vi "Framework Test.vi"() -> ()   [LabVIEW 2017]
uses:
  Builds/Data Sharing Framework/Windows/32/Data Sharing Framework Core/DSF Core.lvlibp/DSF Configuration API/Public/Controls/DSF Direction.ctl
  Builds/Data Sharing Framework/Windows/32/Data Sharing Framework Core/DSF Core.lvlibp/DSF Configuration API/Public/Controls/DSF Timing Info.ctl
  Builds/Data Sharing Framework/Windows/32/Data Sharing Framework Core/DSF Core.lvlibp/DSF Configuration API/Public/Controls/DSF Settings Info.ctl
  Builds/Data Sharing Framework/Windows/32/Data Sharing Framework Core/DSF Core.lvlibp/DSF Configuration API/Public/Controls/DSF Data Type.ctl
  <vilib>/Platform/TimedLoop/XDataNode/timing_clust.ctl
  <vilib>/Platform/TimedLoop/XDataNode/nitl_modes.ctl
  <vilib>/Platform/TimedLoop/XDataNode/wakeup.ctl
  Builds/Data Sharing Framework/Windows/32/Data Sharing Framework Core/DSF Core.lvlibp/Engine/Classes/Debug/FIFO Flags.lvclass
  Builds/Data Sharing Framework/Windows/32/Data Sharing Framework Core/DSF Core.lvlibp/Engine/Classes/Debug/Debug Flags.lvclass
  Builds/Data Sharing Framework/Windows/32/Data Sharing Framework Core/DSF Core.lvlibp/Engine/Classes/Framework/Framework.lvclass
  <vilib>/NI/Memory Manager/Classes/Pointer/Memory.Pointer.lvclass/Memory.Pointer.ctl
  <vilib>/NI/Memory Manager/Classes/Pointer/Memory.Pointer.New.4B.vi
  <vilib>/NI/Memory Manager/Classes/Pointer/Memory.Pointer.Write.0D.U32.vi
  <vilib>/NI/Memory Manager/Classes/Pointer/Memory.Pointer.New.1B.vi
  <vilib>/NI/Memory Manager/Classes/Pointer/Memory.Pointer.Write.0D.Bool.vi
  <vilib>/NI/Memory Manager/Classes/Pointer/Memory.Pointer.New.8B.vi
  <vilib>/NI/Memory Manager/Classes/Pointer/Memory.Pointer.Read.0D.I32.vi
  <vilib>/NI/Memory Manager/Classes/Pointer/Memory.Pointer.Read.0D.U32.vi
  <vilib>/NI/Memory Manager/Classes/Pointer/Memory.Pointer.Read.0D.Bool.vi
  <vilib>/NI/Memory Manager/Classes/Pointer/Memory.Pointer.Write.0D.I32.vi
  <vilib>/NI/Memory Manager/Classes/Pointer/Memory.Pointer.Allocate.vi
  <vilib>/NI/Memory Manager/Classes/Pointer/Memory.Pointer.Write.No Check.0D.U32.vi
  <vilib>/NI/Memory Manager/Classes/Pointer/Memory.Pointer.Parameter Check.Null Pointer.vi
  <vilib>/NI/Memory Manager/Classes/Pointer/Memory.Pointer.Parameter Check.Subset.vi
  <vilib>/NI/Memory Manager/Classes/Pointer/Memory.Pointer.Write.No Check.0D.Bool.vi
  <vilib>/NI/Memory Manager/Classes/Pointer/Memory.Pointer.Read.No Check.0D.I32.vi
  <vilib>/NI/Memory Manager/Classes/Pointer/Memory.Pointer.Read.No Check.0D.U32.vi
  <vilib>/NI/Memory Manager/Classes/Pointer/Memory.Pointer.Read.No Check.0D.Bool.vi
  <vilib>/NI/Memory Manager/Classes/Pointer/Memory.Pointer.Write.No Check.0D.I32.vi
  <vilib>/NI/Memory Manager/Classes/Pointer/Memory.Pointer.Set Address.vi
  <vilib>/NI/Memory Manager/Classes/Pointer/Memory.Pointer.Set Size.vi
  <vilib>/NI/Memory Manager/Classes/Pointer/Memory.Pointer.Set Allocated.vi
  <vilib>/NI/Memory Manager/Classes/Pointer/Memory.Pointer.Errors.vi
  <vilib>/NI/Memory Manager/Classes/Pointer/Memory.Pointer.Errors.Null Pointer.vi
  <vilib>/NI/Memory Manager/Classes/Pointer/Memory.Pointer.Errors.Out of Bounds.vi
  <vilib>/NI/Memory Manager/Classes/Pointer/Memory.Pointer.Errors.Create Error.vi
  <vilib>/NI/Memory Manager/VIs/Source.Write.String.vi
  <vilib>/NI/Memory Manager/Classes/Pointer/Memory.Pointer.Errors.Write Pointer Size.vi
  <vilib>/NI/Memory Manager/VIs/Source.Write.Scalar.Base10.vi
  <vilib>/NI/Memory Manager/VIs/Source.Write.Scalar.Base10 (U64).vi
  <vilib>/NI/Memory Manager/VIs/New Error Cluster Constant.vi
  <vilib>/NI/Memory Manager/VIs/New Error Cluster Constant (512B).vi
  <vilib>/NI/Memory Manager/VIs/Error Cluster.Set Status.vi
  <vilib>/NI/Memory Manager/VIs/Error Cluster.Set Code.vi
  <vilib>/NI/Memory Manager/VIs/Error Cluster.Set VI Source.vi
  <vilib>/NI/Memory Manager/Constants/Memory.Constants.vi
  <vilib>/NI/Memory Manager/Constants/Memory.Constants.Library Name.vi
  <vilib>/NI/Memory Manager/Classes/Pointer/Memory.Pointer.Errors.Get Info.vi
  <vilib>/NI/Memory Manager/Classes/Pointer/Memory.Pointer.lvclass
  <vilib>/platform/TimedLoop/XDataNode/XDataNode.xnode
  <vilib>/Platform/TimedLoop/XDataNode/XDNodeRunTimeDep.lvlib
  Builds/Data Sharing Framework/Windows/32/Data Sharing Framework Core/DSF Core.lvlibp/Shared/Classes/Framework/Framework Configuration.lvclass
  Builds/Data Sharing Framework/Windows/32/Data Sharing Framework Core/DSF Core.lvlibp/Engine/Classes/Status/Framework Status.lvclass
  Builds/Data Sharing Framework/Windows/32/Data Sharing Framework Core/DSF Core.lvlibp/Engine/Classes/Status/Framework Performance.lvclass
  Builds/Data Sharing Framework/Windows/32/Data Sharing Framework Core/DSF Core.lvlibp
panel:
  in  "UDP Rx max size":i32=800
  in  "UDP Rx ports":u16[](array[numeric])=[60000, 60001, 60002, 60003]
  in  "Plugins":T5(array[cluster])=[{"plugin class"="UDP Transceiver", "group configs"=[{"direction"=enum."Tx", "timing"={"priority"=100, "decimation"=1, "offset"=0}, "settings"=[], "transfer configs"=[{"random types?"=FALSE, "non-random type"=enum."DBL", "channel count"=100, "settings"=[{"key"="Destination Address", "value"="localhost"}, {"key"="Destination Port", "value"="60000"}]}]}, {"direction"=enum."Tx", "timing"={"priority"=100, "decimation"=2, "offset"=0}, "settings"=[], "transfer configs"=[{"random types?"=FALSE, "non-random type"=enum."DBL", "channel count"=100, "settings"=[{"key"="Destination Address", "value"="localhost"}, {"key"="Destination Port", "value"="60001"}]}]}, {"direction"=enum."Tx", "timing"={"priority"=100, "decimation"=3, "offset"=0}, "settings"=[], "transfer configs"=[{"random types?"=FALSE, "non-random type"=enum."DBL", "channel count"=100, "settings"=[{"key"="Destination Address", "value"="localhost"}, {"key"="Destination Port", "value"="60002"}]}]}, {"direction"=enum."Tx", "timing"={"priority"=100, "decimation"=4, "offset"=0}, "settings"=[], "transfer configs"=[{"random types?"=FALSE, "non-random type"=enum."DBL", "channel count"=100, "settings"=[{"key"="Destination Address", "value"="localhost"}, {"key"="Destination Port", "value"="60003"}]}]}], "plugin timing"={"priority"=100, "decimation"=1, "offset"=0}, "settings"=[{"key"="Local Port", "value"="50000"}]}]
  in  "Infinite Timeouts":bool=TRUE
  out "Framework Error":errorcluster
  out "Tx duration":u32 format="%d us"
  out "Rx duration":u32 format="%d us"
  out "Actual Frequency":dbl format="%.0pHz"
  in  "Transceiver Count":i32=4
  in  "Configuration Path":path=path "C:/Users/Admin/Desktop/test.dsf"
  out "Framework Iteration":i32 format="%d cycles"
  out "Actual Period":u32 format="%d us"
  in  "Target PCL Period":u32=10000 caption="Target Period" format="%d us"
  in  "stop":bool
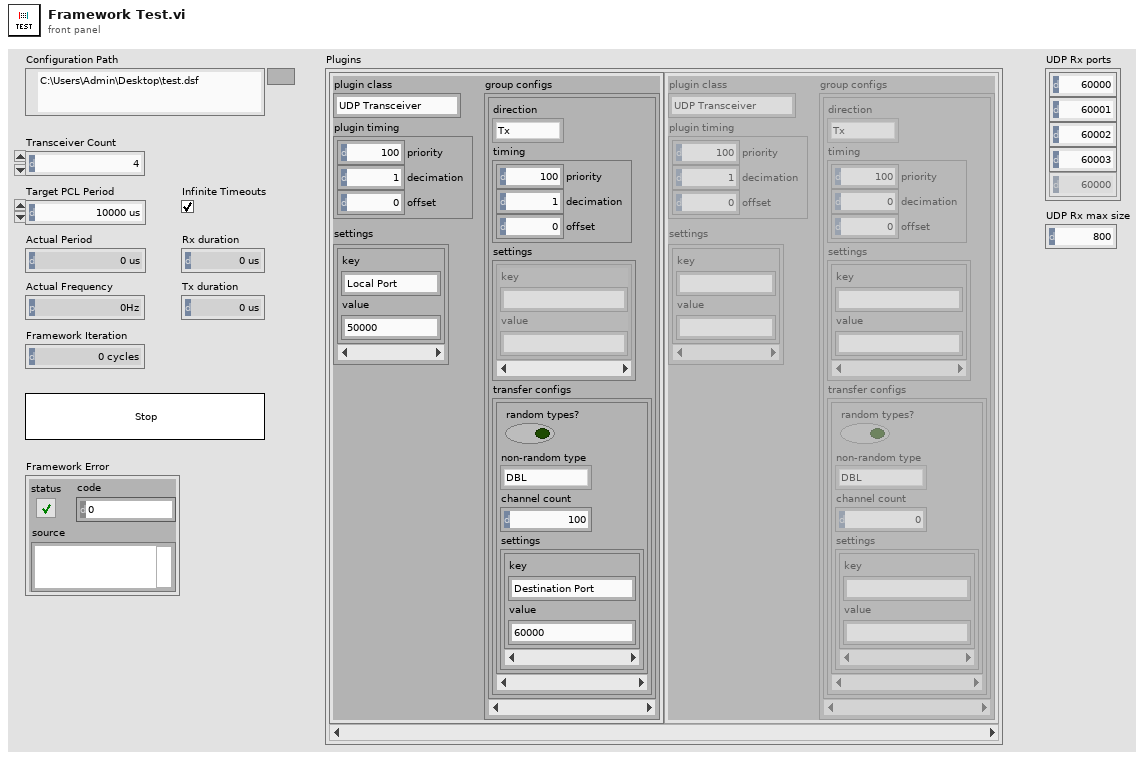
[diagram p1: front panel]
types:
  T1 = typedef "DSF Core.lvlibp/DSF Direction.ctl" = enum8{"Tx", "Rx"}
  T2 = typedef "DSF Core.lvlibp/DSF Timing Info.ctl" = cluster{"priority":u64, "decimation":u64, "offset":u64}
  T3 = typedef "DSF Core.lvlibp/DSF Settings Info.ctl" = cluster{"key":string, "value":string}[]
  T4 = typedef "DSF Core.lvlibp/DSF Data Type.ctl" = enum8{"Bool", "SGL", "DBL", "I8", "I16", "I32", "I64", "U8", "U16", "U32", "U64"}
  T5 = cluster{"plugin class":string, "group configs":cluster{"direction":T1, "timing":T2, "settings":T3, "transfer configs":cluster{"random types?":bool, "non-random type":T4, "channel count":i32, "settings":T3}[]}[], "plugin timing":T2, "settings":T3}[]
  T6 = typedef "DSF Core.lvlibp/DSF Engine Framework Configuration.ctl" = cluster{"Plugins":T7[]}
  T7 = typedef "DSF Core.lvlibp/DSF Engine Plugin Configuration.ctl" = cluster{"name":string, "class":string, "cycle timing":T2, "Transfer Groups":T8[], "settings":T3}
  T8 = typedef "DSF Core.lvlibp/DSF Engine Transfer Group Configuration.ctl" = cluster{"name":string, "direction":T1, "cycle timing":T2, "Transfers":T9[], "settings":T3}
  T9 = typedef "DSF Core.lvlibp/DSF Engine Transfer Configuration.ctl" = cluster{"name":string, "byte order":T10, "channel configurations":T11[], "settings":T3}
  T10 = typedef "DSF Core.lvlibp/DSF Byte Order.ctl" = enum8{"big-endian", "little-endian"}
  T11 = typedef "DSF Core.lvlibp/DSF Engine Channel Configuration.ctl" = cluster{"engine offset":u64, "name":string, "data type":T4, "count":u64, "buffer offset":u64, "settings":T3}
  T12 = typedef "XDNodeRunTimeDep.lvlib/timing_clust.ctl" = cluster{"Expected End [f-1]":u64, "Actual End [f-1]":u64, "Finished Late? [f-1]":bool, "Expected End [i-1]":u64, "Actual End [i-1]":u64, "Finished Late? [i-1]":bool, "Expected Start [i]":u64, "Actual Start [i]":u64, "Expected Start [f]":u64, "Actual Start [f]":u64, "Source Name":string, "Structure Name":string, "Period":i64, "Deadline":i64, "Offset":i64, "Start":i64, "Priority":i32, "Timeout":i32, "Mode":T13, "Wakeup Reason":T14, "Error":errorcluster, "Source Type":string, "Secondary Source Type":string, "Global End Time":u64, "Global Start Time":u64, "Frame Duration":u64, "Iteration Duration":u64, "Assigned CPU":i32, "I/O Scan Engine Mode":u32}
  T13 = typedef "XDNodeRunTimeDep.lvlib/nitl_modes.ctl" = enum32{"No Change", "Process missed periods, maintain original phase", "Discard missed periods, maintain original phase", "Process missed periods, ignore original phase", "Discard missed periods, ignore original phase"}
  T14 = typedef "XDNodeRunTimeDep.lvlib/wakeup.ctl" = enum32{"Normal", "Aborted", "Asynchronous wakeup", "Timing source error", "Timed loop error", "Timeout"}
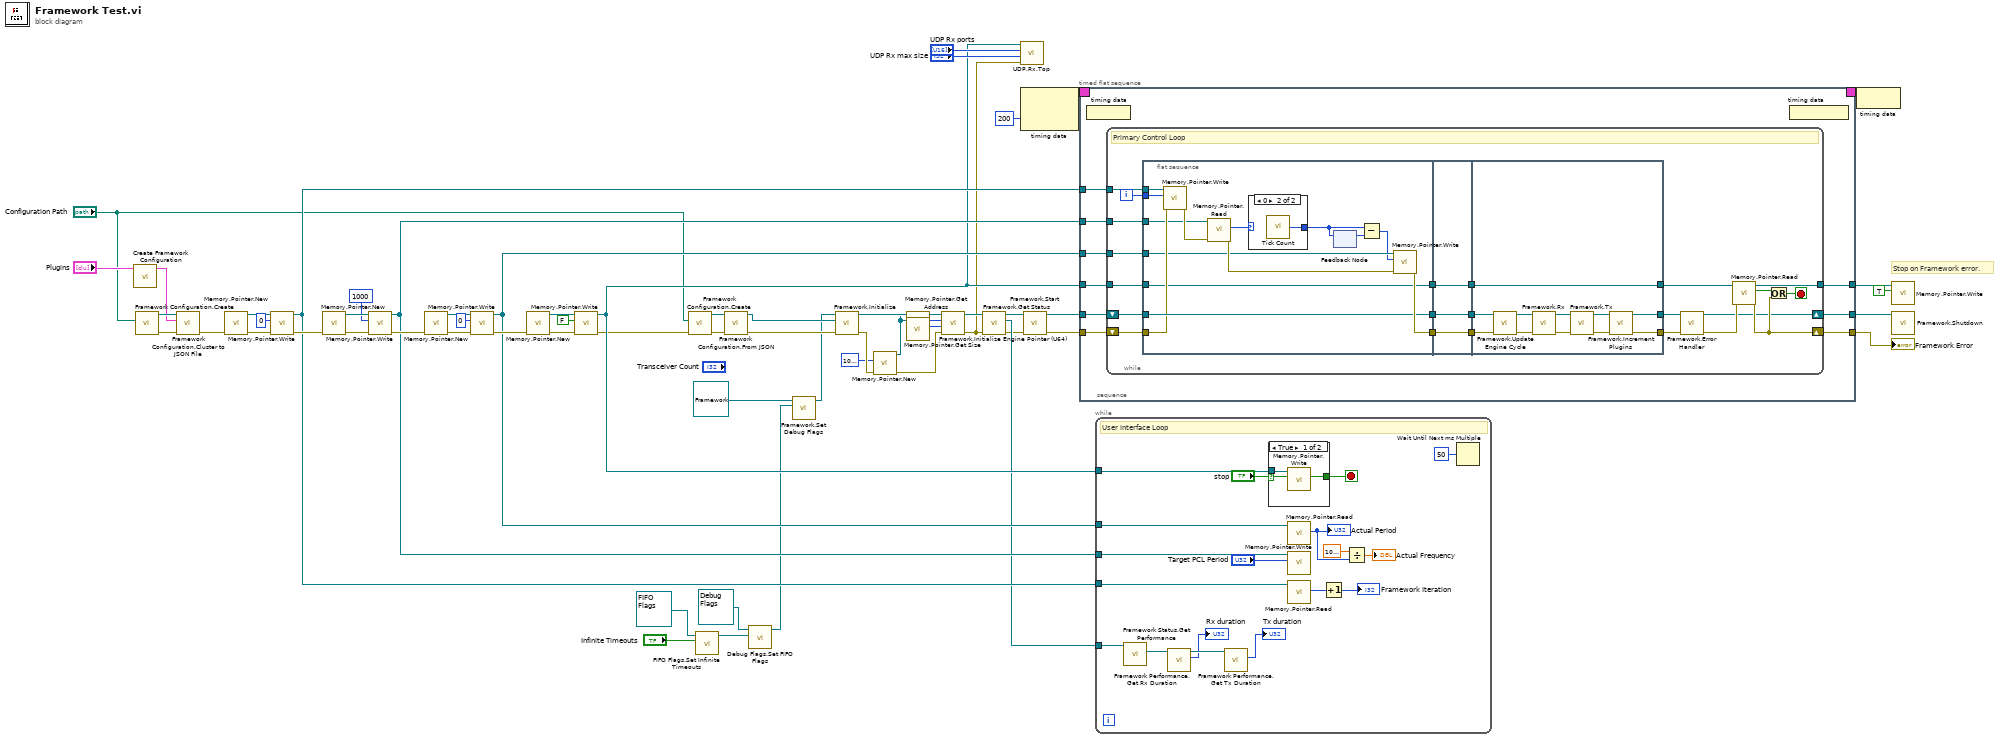
[diagram p0: block diagram]
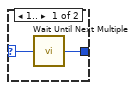
[diagram p2: hidden frame]
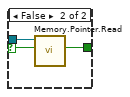
[diagram p3: hidden frame]
diagram:
  # "Stop on Framework error."
  n1 = call "Create Framework Configuration.vi"("Plugins"="Plugins") -> ("Framework Configuration"=w28:T6)  [unwired: 10 in]
  n2 = call "Framework Configuration.Create.vi"("configuration path"="Configuration Path") -> ("error out"=w30:errorcluster, "Framework Configuration"=w31:refnum<class "Framework Configuration.lvclass">)  [unwired: 9 in]
  n3 = call "Framework Configuration.Cluster to JSON File.vi"("error in (no error)"=w30, "Framework Configuration"=w28, "Framework Configuration in"=w31) -> ("error out"=w29:errorcluster)  [unwired: 7 in, 1 out]
  n4 = call-poly <vilib>:"Memory.Pointer.New.vi"("error in (no error)"=w29) -> ("error out"=w44:errorcluster, "Pointer"=w45:refnum<class "Memory.Pointer.lvclass">)  [unwired: 9 in]
  n5 = call-poly <vilib>:"Memory.Pointer.Write.vi"("error in (no error)"=w44, "value"=u32 0, "Pointer in"=w45) -> ("error out"=w43:errorcluster, "Pointer out"=w42:refnum<class "Memory.Pointer.lvclass">)  [unwired: 5 in, 2 out]
  n6 = call-poly <vilib>:"Memory.Pointer.New.vi"("error in (no error)"=w43) -> ("error out"=w51:errorcluster, "Pointer"=w52:refnum<class "Memory.Pointer.lvclass">)  [unwired: 9 in]
  n7 = call-poly <vilib>:"Memory.Pointer.Write.vi"("error in (no error)"=w51, "value"=u32 1000, "Pointer in"=w52) -> ("error out"=w50:errorcluster, "Pointer out"=w46:refnum<class "Memory.Pointer.lvclass">)  [unwired: 5 in, 2 out]
  n8 = call-poly <vilib>:"Memory.Pointer.New.vi"("error in (no error)"=w50) -> ("error out"=w49:errorcluster, "Pointer"=w53:refnum<class "Memory.Pointer.lvclass">)  [unwired: 9 in]
  n9 = call-poly <vilib>:"Memory.Pointer.Write.vi"("error in (no error)"=w49, "value"=u32 0, "Pointer in"=w53) -> ("error out"=w48:errorcluster, "Pointer out"=w47:refnum<class "Memory.Pointer.lvclass">)  [unwired: 5 in, 2 out]
  n10 = call-poly <vilib>:"Memory.Pointer.New.vi"("error in (no error)"=w48) -> ("error out"=w56:errorcluster, "Pointer"=w55:refnum<class "Memory.Pointer.lvclass">)  [unwired: 9 in]
  n11 = call-poly <vilib>:"Memory.Pointer.Write.vi"("error in (no error)"=w56, "value"=FALSE, "Pointer in"=w55) -> ("error out"=w27:errorcluster, "Pointer out"=w34:refnum<class "Memory.Pointer.lvclass">)  [unwired: 5 in, 2 out]
  n12 = call "Framework Configuration.Create.vi"("error in (no error)"=w27, "configuration path"="Configuration Path") -> ("error out"=w24:errorcluster, "Framework Configuration"=w25:refnum<class "Framework Configuration.lvclass">)  [unwired: 8 in]
  n13 = call "FIFO Flags.Set Infinite Timeouts.vi"("infinite timeouts"="Infinite Timeouts", "FIFO Debug Flags in"=refnum<class "FIFO Flags.lvclass"> refnum ("DSF Core.lvlibp:FIFO Flags.lvclass")) -> ("FIFO Debug Flags out"=w19:refnum<class "FIFO Flags.lvclass">)  [unwired: 9 in]
  n14 = call "Framework Configuration.From JSON.vi"("error in (no error)"=w24, "Framework Configuration in"=w25) -> ("error out"=w23:errorcluster, "Framework Configuration out"=w22:refnum<class "Framework Configuration.lvclass">)  [unwired: 8 in]
  n15 = call "Debug Flags.Set FIFO Flags.vi"("FIFO"=w19, "Debug Flags in"=refnum<class "Debug Flags.lvclass"> refnum ("DSF Core.lvlibp:Debug Flags.lvclass")) -> ("Debug Flags out"=w16:refnum<class "Debug Flags.lvclass">)  [unwired: 9 in]
  n16 = call "Framework.Set Debug Flags.vi"("Debug Flags"=w16, "Framework in"=refnum<class "Framework.lvclass"> refnum ("DSF Core.lvlibp:Framework")) -> ("Framework out"=w15:refnum<class "Framework.lvclass">)  [unwired: 9 in]
  n17 = call "Framework.Initialize.vi"("error in (no error)"=w23, "Framework Configuration"=w22, "Framework type"=w15) -> ("error out"=w6:errorcluster, "Framework out"=w9:refnum<class "Framework.lvclass">)  [unwired: 7 in]
  n18 = call-poly <vilib>:"Memory.Pointer.New.vi"("error in (no error)"=w6, "count (1)"=u64 1000000 ("channel count")) -> ("error out"=w5:errorcluster, "Pointer"=w2:refnum<class "Memory.Pointer.lvclass">)  [unwired: 8 in]
  n19 = call <vilib>:"Memory.Pointer.Get Address.vi"("Pointer in"=w2) -> ("address"=w4:u64)  [unwired: 9 in, 1 out]
  n20 = call <vilib>:"Memory.Pointer.Get Size.vi"("Pointer in"=w2) -> ("size"=w3:u64)  [unwired: 9 in, 1 out]
  n21 = call "Framework.Initialize Engine Pointer (U64).vi"("error in (no error)"=w5, "size"=w3, "address"=w4, "Framework in"=w9) -> ("error out"=w7:errorcluster, "Framework out"=w8:refnum<class "Framework.lvclass">)  [unwired: 6 in]
  n22 = call "Framework.Get Status.vi"("Framework in"=w8) -> ("Status"=w11:refnum<class "Framework Status.lvclass">, "Framework out"=w12:refnum<class "Framework.lvclass">)  [unwired: 9 in]
  n23 = call "UDP.Rx.Top.vi"("error in (no error)"=w7, "max size (800)"="UDP Rx max size", "ports"="UDP Rx ports", "Stop Pointer"=w34) -> ()  [unwired: 7 in, 1 out]
  n24 = node-c288(200 ("Priority")) -> (w58:T12)  [unwired: 1 in]
  n25 = call "Framework.Start.vi"("error in (no error)"=w7, "Framework in"=w12) -> ("error out"=w13:errorcluster, "Framework out"=w14:refnum<class "Framework.lvclass">)  [unwired: 8 in]
  n26 = timed-sequence {
    timing: w58 -> [_]
    timing-out: [_] -> w57
    tunnel: w14 -> [w68]
    tunnel: w13 -> [w67]
    tunnel: [w66] -> w10
    tunnel: [w65] -> w59
    tunnel: w34 -> [w64]
    tunnel: w46 -> [w63]
    tunnel: w47 -> [w62]
    tunnel: w42 -> [w61]
    tunnel: [w60] -> w33
    n27 = timed-flat-sequence {
      tunnel: w68 -> [w77]
      tunnel: w67 -> [w76]
      tunnel: [w75] -> w66
      tunnel: [w74] -> w65
      tunnel: w64 -> [w73]
      tunnel: w63 -> [w72]
      tunnel: w62 -> [w71]
      tunnel: w61 -> [w70]
      tunnel: [w69] -> w60
      n28 = node-c288() -> ()  [unwired: 1 in]
      n29 = while {
        shift-right: [w78] -> w75
        shift-left: w77 -> [w98]
        shift-right: [w92] -> w74
        shift-left: w76 -> [w99]
        tunnel: w73 -> [w97]
        tunnel: w72 -> [w95]
        tunnel: w71 -> [w94]
        tunnel: w70 -> [w90]
        tunnel: [w82] -> w69
        i -> [w89]
        stop <- w91 stop-if-true
        # "Primary Control Loop"
        n30 = flat-sequence {
          tunnel: w99 -> [w108]
          tunnel: w98 -> [w111]
          tunnel: w97 -> [w104]
          tunnel: [w112] -> w88
          tunnel: [w111] -> w86
          tunnel: [w104] -> w84
          tunnel: w95 -> [w106]
          tunnel: w94 -> [w105]
          tunnel: w90 -> [w109]
          tunnel: w89 -> [w102]
          tunnel: w88 -> [w119]
          tunnel: [w119] -> w87
          tunnel: w86 -> [w118]
          tunnel: [w118] -> w85
          tunnel: w84 -> [w117]
          tunnel: [w117] -> w83
          tunnel: w87 -> [w128]
          tunnel: w85 -> [w129]
          tunnel: w83 -> [w130]
          tunnel: [w130] -> w96
          tunnel: [w121] -> w80
          tunnel: [w120] -> w81
          frame #0 {
            n31 = call-poly <vilib>:"Memory.Pointer.Write.vi"("error in (no error)"=w108, "value"=w102, "Pointer in"=w109) -> ("error out"=w107:errorcluster)  [unwired: 5 in, 3 out]
            n32 = call-poly <vilib>:"Memory.Pointer.Read.vi"("error in (no error)"=w107, "Pointer in"=w106) -> ("error out"=w110:errorcluster, "value out"=w100:u32)  [unwired: 6 in, 2 out]
            n33 = case shown="0" w100 {
              selector: w100 -> [w114 _]
              tunnel: [w115 w116] -> w103
              frame 1.. {
                n34 = call "Wait Until Next Multiple"("Count(uSec)"=w114) -> ("Tick Count(uSec)"=w115:u32)
              }
              frame 0 {
                n35 = call "Tick Count"() -> ("Tick Count(uSec)"=w116:u32)
              }
            }
            n36 = feedback #1() -> (w113:u32)  [unwired: 1 in]
            n37 = feedback-in #1(w103) -> ()
            n38 = Subtract(x=w103, y=w113) -> (x-y=w101:u32)
            n39 = call-poly <vilib>:"Memory.Pointer.Write.vi"("error in (no error)"=w110, "value"=w101, "Pointer in"=w105) -> ("error out"=w112:errorcluster)  [unwired: 5 in, 3 out]
          }
          frame #1 {
          }
          frame #2 {
            n40 = call-dynamic "Framework.Update Engine Cycle.vi"("error in (no error)"=w128, "Framework in"=w129) -> ("error out"=w126:errorcluster, "Framework out"=w127:refnum<class "Framework.lvclass">)  [unwired: 8 in]
            n41 = call "Framework.Rx.vi"("error in (no error)"=w126, "Framework in"=w127) -> ("error out"=w124:errorcluster, "Framework out"=w125:refnum<class "Framework.lvclass">)  [unwired: 8 in]
            n42 = call "Framework.Tx.vi"("error in (no error)"=w124, "Framework in"=w125) -> ("error out"=w123:errorcluster, "Framework out"=w122:refnum<class "Framework.lvclass">)  [unwired: 8 in]
            n43 = call "Framework.Increment Plugins.vi"("error in (no error)"=w123, "Framework in"=w122) -> ("error out"=w120:errorcluster, "Framework out"=w121:refnum<class "Framework.lvclass">)  [unwired: 8 in]
          }
        }
        n44 = call "Framework.Error Handler.vi"("error in (no error)"=w81, "Framework in"=w80) -> ("error out"=w79:errorcluster, "Framework out"=w78:refnum<class "Framework.lvclass">)  [unwired: 8 in]
        n45 = call-poly <vilib>:"Memory.Pointer.Read.vi"("error in (no error)"=w79, "Pointer in"=w96) -> ("error out"=w92:errorcluster, "value out"=w93:bool, "Pointer out"=w82:refnum<class "Memory.Pointer.lvclass">)  [unwired: 6 in, 1 out]
        n46 = Or(x=w93, y=w92) -> (x .or. y?=w91:bool)
      }
      n47 = node-c288() -> ()  [unwired: 1 out]
    }
  }
  "Framework Error" <- w59
  n48 = while {
    tunnel: w34 -> [w149]
    tunnel: w47 -> [w146]
    tunnel: w46 -> [w147]
    tunnel: w42 -> [w143]
    tunnel: w11 -> [w137]
    stop <- w150 stop-if-true
    # "User Interface Loop"
    n49 = call "Framework Status.Get Performance.vi"("Framework Status in"=w137) -> ("Framework Performance"=w136:refnum<class "Framework Performance.lvclass">)  [unwired: 9 in, 1 out]
    n50 = call "Framework Performance.Get Rx Duration.vi"("Framework Performance in"=w136) -> ("rx duration"=→"Rx duration":u32, "Framework Performance out"=w135:refnum<class "Framework Performance.lvclass">)  [unwired: 8 in, 1 out]
    n51 = call "Framework Performance.Get Tx Duration.vi"("Framework Performance in"=w135) -> ("tx duration"=→"Tx duration":u32)  [unwired: 8 in, 2 out]
    n52 = case shown="True" "stop" {
      selector: "stop" -> [w151 w154]
      tunnel: [w153 w156] -> w150
      tunnel: w149 -> [w152 w155]
      frame True {
        n53 = call-poly <vilib>:"Memory.Pointer.Write.vi"("value"=w151, "Pointer in"=w152) -> ("value"=w153:bool)  [unwired: 6 in, 3 out]
      }
      frame False {
        n54 = call-poly <vilib>:"Memory.Pointer.Read.vi"("value in"=w154, "Pointer in"=w155) -> ("value out"=w156:bool)  [unwired: 6 in, 3 out]
      }
    }
    n55 = call-poly <vilib>:"Memory.Pointer.Read.vi"("Pointer in"=w146) -> ("value out"=w141:u32)  [unwired: 7 in, 3 out]
    "Actual Period" <- w141
    n56 = call-poly <vilib>:"Memory.Pointer.Write.vi"("value"="Target PCL Period", "Pointer in"=w147) -> ()  [unwired: 6 in, 4 out]
    n57 = call-poly <vilib>:"Memory.Pointer.Read.vi"("Pointer in"=w143) -> ("value out"=w140:i32)  [unwired: 7 in, 3 out]
    n58 = Increment(x=w140) -> (x+1=→"Framework Iteration":i32)
    n59 = Divide(x=1000000.0, y=w141) -> (x/y=→"Actual Frequency":dbl)
    n60 = Wait Until Next ms Multiple(millisecond multiple=u32 50 ("milliseconds to wait")) -> ()  [unwired: 1 out]
  }
  n61 = node-c288(w57) -> ()
  n62 = call-poly <vilib>:"Memory.Pointer.Write.vi"("value"=TRUE, "Pointer in"=w33) -> ()  [unwired: 6 in, 4 out]
  n63 = call "Framework.Shutdown.vi"("Framework in"=w10) -> ()  [unwired: 9 in, 2 out]
